vi "client example -dual tone - digital.vi"() -> ()   [LabVIEW 2021]
uses:
  controls/digital protocol settings.ctl
  <vilib>/PDM Acquisition Toolkit/host/Classes/Session/Controls/Logic Levels.ctl
  <vilib>/PDM Acquisition Toolkit/shared/controls/PCM Data Format Configuration.ctl
  <vilib>/PDM Acquisition Toolkit/shared/controls/Digital Edge.ctl
  <vilib>/PDM Acquisition Toolkit/shared/controls/PCM Bit Endianness.ctl
  <vilib>/PDM Acquisition Toolkit/shared/controls/PCM Data Justification.ctl
  <vilib>/PDM Acquisition Toolkit/shared/controls/clock mode.ctl
  <vilib>/PDM Acquisition Toolkit/shared/controls/PCM Frame Sync Control.ctl
  controls/generation status.ctl
  controls/dual tone properties.ctl
  controls/dual tone types.ctl
  AudioGeneration/Configure - Digital.vi
  AudioGeneration/AudioGeneration.lvclass
  <vilib>/PDM Acquisition Toolkit/host/Classes/Session/DecoderSession.lvclass
  <vilib>/PDM Acquisition Toolkit/shared/PDM Shared.lvlib
  controls/AudioGenTypeDefs.lvlib
panel:
  in  "dual tone properties":T1
  in  "Update":bool
  out "status":T3
  in  "stop":bool
  in  "digital protocol settings":T4={"logic level"=enum."3.3 V", "PCM Data Configuration"={"Frame Sync Edge for Channel 0"=enum."Rising", "Channel Count Per Frame"=2, "Channel Length"=32, "Bit Depth"=24, "Channel 0 Offset"=1, "Endianness"=enum."MSB First", "Data Justification"=enum."Left Justified"}, "bit clock rate"=3072000.0, "master clock rate"=12288000.0, "clock mode"=enum."DDS", "Frame Sync Clock Control"={"Frame Length"=64, "Frame Sync Pulse Width"=32, "Bit Clock Edge  Sync"=enum."Rising"}} {"master clock rate" format="%.4p"; "bit clock rate" format="%.4p"}
  in  "master clock channel list":string="7821\\PCMo 0"
  in  "data channel list":string="7821\\PCMo 8"
  out "error out":errorcluster
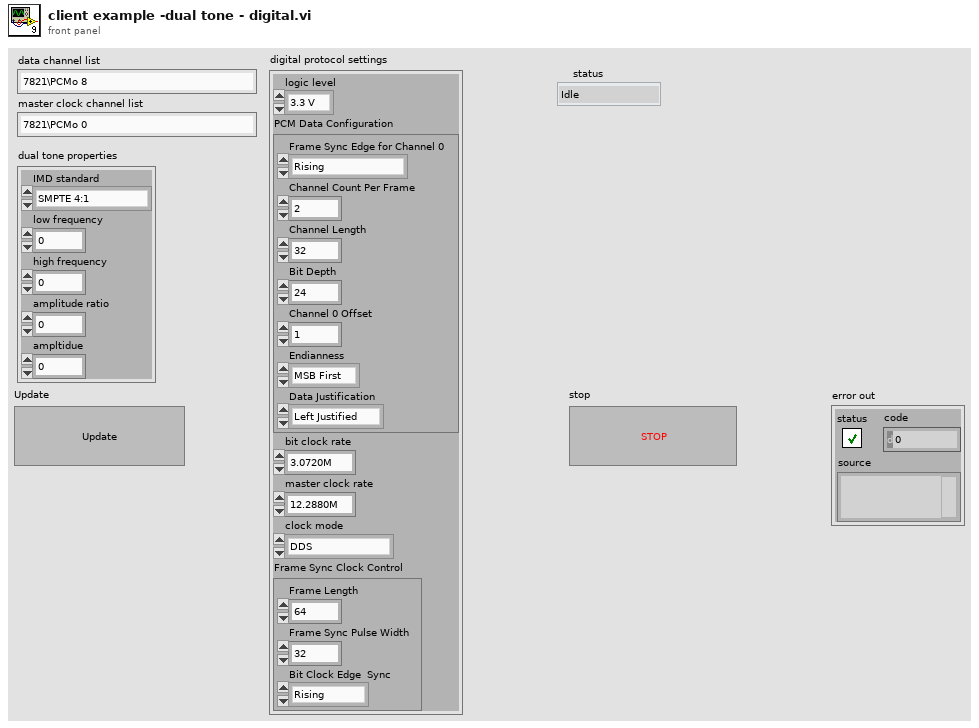
[diagram p1: front panel]
types:
  T1 = typedef "AudioGenTypeDefs.lvlib/dual tone properties.ctl" = cluster{"IMD standard":T2, "low frequency":dbl, "high frequency":dbl, "amplitude ratio":dbl, "ampltidue":dbl}
  T2 = typedef "AudioGenTypeDefs.lvlib/dual tone types.ctl" = enum32{"SMPTE 4:1", "DIN", "CCIF 11k-12k", "CCIF 19k-20k", "Custom"}
  T3 = typedef "AudioGenTypeDefs.lvlib/generation status.ctl" = enum16{"Idle", "Committed", "Active"}
  T4 = typedef "AudioGenTypeDefs.lvlib/digital protocol settings.ctl" = cluster{"logic level":T5, "PCM Data Configuration":T6, "bit clock rate":sgl, "master clock rate":sgl, "clock mode":T10, "Frame Sync Clock Control":T11}
  T5 = typedef "PDM Acquisition Class Library.lvlib/DecoderSession.lvclass/Logic Levels.ctl" = enum16{"3.3 V", "1.8 V", "1.2 V"}
  T6 = typedef "PDM Shared.lvlib/PCM Data Format Configuration.ctl" = cluster{"Frame Sync Edge for Channel 0":T7, "Channel Count Per Frame":u8, "Channel Length":u16, "Bit Depth":u8, "Channel 0 Offset":u16, "Endianness":T8, "Data Justification":T9}
  T7 = typedef "PDM Shared.lvlib/Digital Edge.ctl" = enum8{"Rising", "Falling"}
  T8 = typedef "PDM Shared.lvlib/PCM Bit Endianness.ctl" = enum16{"MSB First", "LSB First"}
  T9 = typedef "PDM Shared.lvlib/PCM Data Justification.ctl" = enum16{"Left Justified", "Right Justified"}
  T10 = typedef "PDM Shared.lvlib/clock mode.ctl" = enum16{"divided clock", "DDS"}
  T11 = typedef "PDM Shared.lvlib/PCM Frame Sync Control.ctl" = cluster{"Frame Length":u16, "Frame Sync Pulse Width":u16, "Bit Clock Edge  Sync":T7}
  T12 = typedef "AudioGenTypeDefs.lvlib/signal settings.ctl" = cluster{"signal type":T13, "properties":string, "output level units":T14}
  T13 = typedef "AudioGenTypeDefs.lvlib/signal type.ctl" = enum16{"Sine", "Dual Tone"}
  T14 = typedef "audio controls.lvlib/digital output level units.ctl" = enum32{"% FS", "dBFS", "V"}
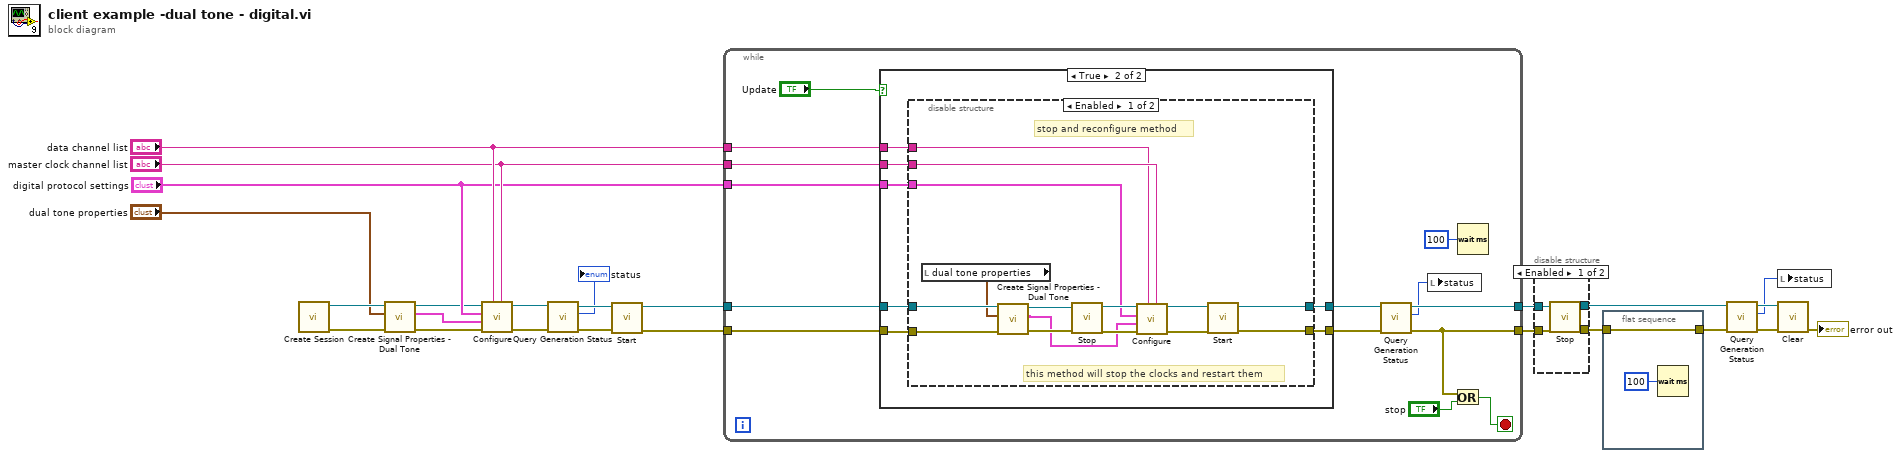
[diagram p0: block diagram]
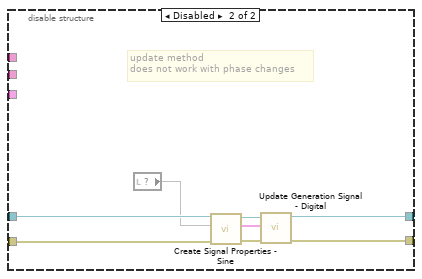
[diagram p4: hidden frame]
diagram:
  n1 = call "Create Session.vi"() -> ("error out"=w5:errorcluster, "session out"=w4:refnum<class "AudioGeneration.lvclass">)  [unwired: 10 in]
  n2 = call "Create Signal Properties - Dual Tone.vi"("error in (no error)"=w5, "dual tone properties"="dual tone properties", "AudioGeneration in"=w4) -> ("error out"=w6:errorcluster, "signal settings"=w2:T12, "AudioGeneration out"=w3:refnum<class "AudioGeneration.lvclass">)  [unwired: 6 in]
  n3 = call-poly "Configure.vi"("master clock channel list"="master clock channel list", "data channel list"="data channel list", "error in (no error)"=w6, "signal settings"=w2, "digital protocol settings"="digital protocol settings", "AudioGeneration in"=w3) -> ("error out"=w22:errorcluster, "AudioGeneration out"=w19:refnum<class "AudioGeneration.lvclass">)  [unwired: 4 in]
  n4 = call "Query Generation Status.vi"("error in (no error)"=w22, "AudioGeneration in"=w19) -> ("error out"=w21:errorcluster, "status"=→"status":T3, "AudioGeneration out"=w20:refnum<class "AudioGeneration.lvclass">)  [unwired: 5 in, 2 out]
  n5 = call "Start.vi"("error in (no error)"=w21, "AudioGeneration in"=w20) -> ("error out"=w16:errorcluster, "AudioGeneration out"=w17:refnum<class "AudioGeneration.lvclass">)  [unwired: 8 in]
  n6 = while {
    tunnel: [w36] -> w24
    tunnel: [w35] -> w23
    tunnel: w17 -> [w32]
    tunnel: w16 -> [w31]
    tunnel: "data channel list" -> [w28]
    tunnel: "master clock channel list" -> [w27]
    tunnel: "digital protocol settings" -> [w26]
    stop <- w38 stop-if-true
    n7 = case shown="True" "Update" {
      tunnel: w32 -> [w41 w46]
      tunnel: w31 -> [w40 w45]
      tunnel: [w41 w48] -> w30
      tunnel: [w40 w47] -> w29
      tunnel: w28 -> [_ w43]
      tunnel: w27 -> [_ w44]
      tunnel: w26 -> [_ w42]
      frame False {
      }
      frame True {
        n8 = disable-structure shown="Enabled" {
          disable-tunnel: [w55 w71] -> w48
          disable-tunnel: [w56 w70] -> w47
          disable-tunnel: w46 -> [w63 w69]
          disable-tunnel: w45 -> [w62 w64]
          disable-tunnel: w44 -> [w53 _]
          disable-tunnel: w43 -> [w52 _]
          disable-tunnel: w42 -> [w51 _]
          frame Enabled {
            # "this method will stop the clocks and restart them"
            # "stop and reconfigure method"
            n9 = local read "dual tone properties"() -> (w49:T1)
            n10 = call "Create Signal Properties - Dual Tone.vi"("error in (no error)"=w62, "dual tone properties"=w49, "AudioGeneration in"=w63) -> ("error out"=w60:errorcluster, "signal settings"=w50:T12, "AudioGeneration out"=w61:refnum<class "AudioGeneration.lvclass">)  [unwired: 6 in]
            n11 = call "Stop.vi"("error in (no error)"=w60, "AudioGeneration in"=w61) -> ("error out"=w58:errorcluster, "AudioGeneration out"=w59:refnum<class "AudioGeneration.lvclass">)  [unwired: 8 in]
            n12 = call-poly "Configure.vi"("master clock channel list"=w53, "data channel list"=w52, "error in (no error)"=w58, "signal settings"=w50, "digital protocol settings"=w51, "AudioGeneration in"=w59) -> ("error out"=w57:errorcluster, "AudioGeneration out"=w54:refnum<class "AudioGeneration.lvclass">)  [unwired: 4 in]
            n13 = call "Start.vi"("error in (no error)"=w57, "AudioGeneration in"=w54) -> ("error out"=w56:errorcluster, "AudioGeneration out"=w55:refnum<class "AudioGeneration.lvclass">)  [unwired: 8 in]
          }
          frame Disabled {
            # "update method\ndoes not work with phase changes"
            n14 = local read item#-1() -> (w65)
            n15 = call "Create Signal Properties - Sine.vi"("error in (no error)"=w64, "sine wave properties"=w65, "AudioGeneration in"=w69) -> ("error out"=w67:errorcluster, "signal settings"=w66:T12, "AudioGeneration out"=w68:refnum<class "AudioGeneration.lvclass">)  [unwired: 6 in]
            n16 = call "Update Generation Signal - Digital.vi"("error in (no error)"=w67, "signal settings"=w66, "AudioGeneration in"=w68) -> ("error out"=w70:errorcluster, "AudioGeneration out"=w71:refnum<class "AudioGeneration.lvclass">)  [unwired: 7 in]
          }
        }
      }
    }
    n17 = call "Query Generation Status.vi"("error in (no error)"=w29, "AudioGeneration in"=w30) -> ("error out"=w35:errorcluster, "status"=w34:T3, "AudioGeneration out"=w36:refnum<class "AudioGeneration.lvclass">)  [unwired: 5 in, 2 out]
    n18 = local write "status"(w34) -> ()
    n19 = Or(x=w35, y="stop") -> (x .or. y?=w38:bool)
    n20 = Wait (ms)(milliseconds to wait=u32 100) -> ()  [unwired: 1 out]
  }
  n21 = disable-structure shown="Enabled" {
    disable-tunnel: w24 -> [w75 w77]
    disable-tunnel: w23 -> [w74 w76]
    disable-tunnel: [w73 w77] -> w15
    disable-tunnel: [w72 w76] -> w11
    frame Enabled {
      n22 = call "Stop.vi"("error in (no error)"=w74, "AudioGeneration in"=w75) -> ("error out"=w72:errorcluster, "AudioGeneration out"=w73:refnum<class "AudioGeneration.lvclass">)  [unwired: 8 in]
    }
    frame Disabled {
    }
  }
  n23 = flat-sequence {
    tunnel: w11 -> [w79]
    tunnel: [w79] -> w10
    frame #0 {
      n24 = Wait (ms)(milliseconds to wait=u32 100) -> ()  [unwired: 1 out]
    }
  }
  n25 = call "Query Generation Status.vi"("error in (no error)"=w10, "AudioGeneration in"=w15) -> ("error out"=w13:errorcluster, "status"=w12:T3, "AudioGeneration out"=w14:refnum<class "AudioGeneration.lvclass">)  [unwired: 5 in, 2 out]
  n26 = local write "status"(w12) -> ()
  n27 = call "Clear.vi"("error in (no error)"=w13, "AudioGeneration in"=w14) -> ("error out"=→"error out":errorcluster)  [unwired: 9 in]
